vi "BRig_RT__Case_Exp__State_RewardPre__v11.vi"(0 "input_dataCurrent":u16[](array[numeric]), 7 "input_dataExp":u16[](array[numeric]), 9 "input_dataBlock":u16[][](array[numeric]), 11 "input_dataTrial":u16[][](array[numeric]), 12 "input_dataLC":u16[](array[numeric])) -> (1 "output_T_Reward":u16, 2 "output_c_nReward_total_R":u16, 3 "output_c_nReward_total_L":u16, 4 "output_dataCurrent":u16[](array[numeric]), 6 "output_DAB_L=L":bool, 8 "output_DAB_R=HighPorb":bool, 10 "output_dataBlock":u16[][](array[numeric]), 13 "output_c_nReward_total":u16, 14 "output_nReward":u16, 15 "output_dataTrial":u16[][](array[numeric]))   [LabVIEW 2014]
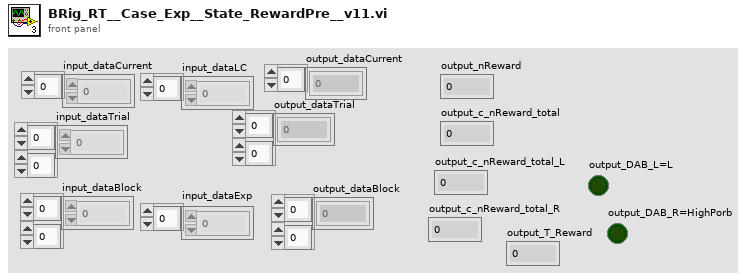
[diagram p1: front panel]
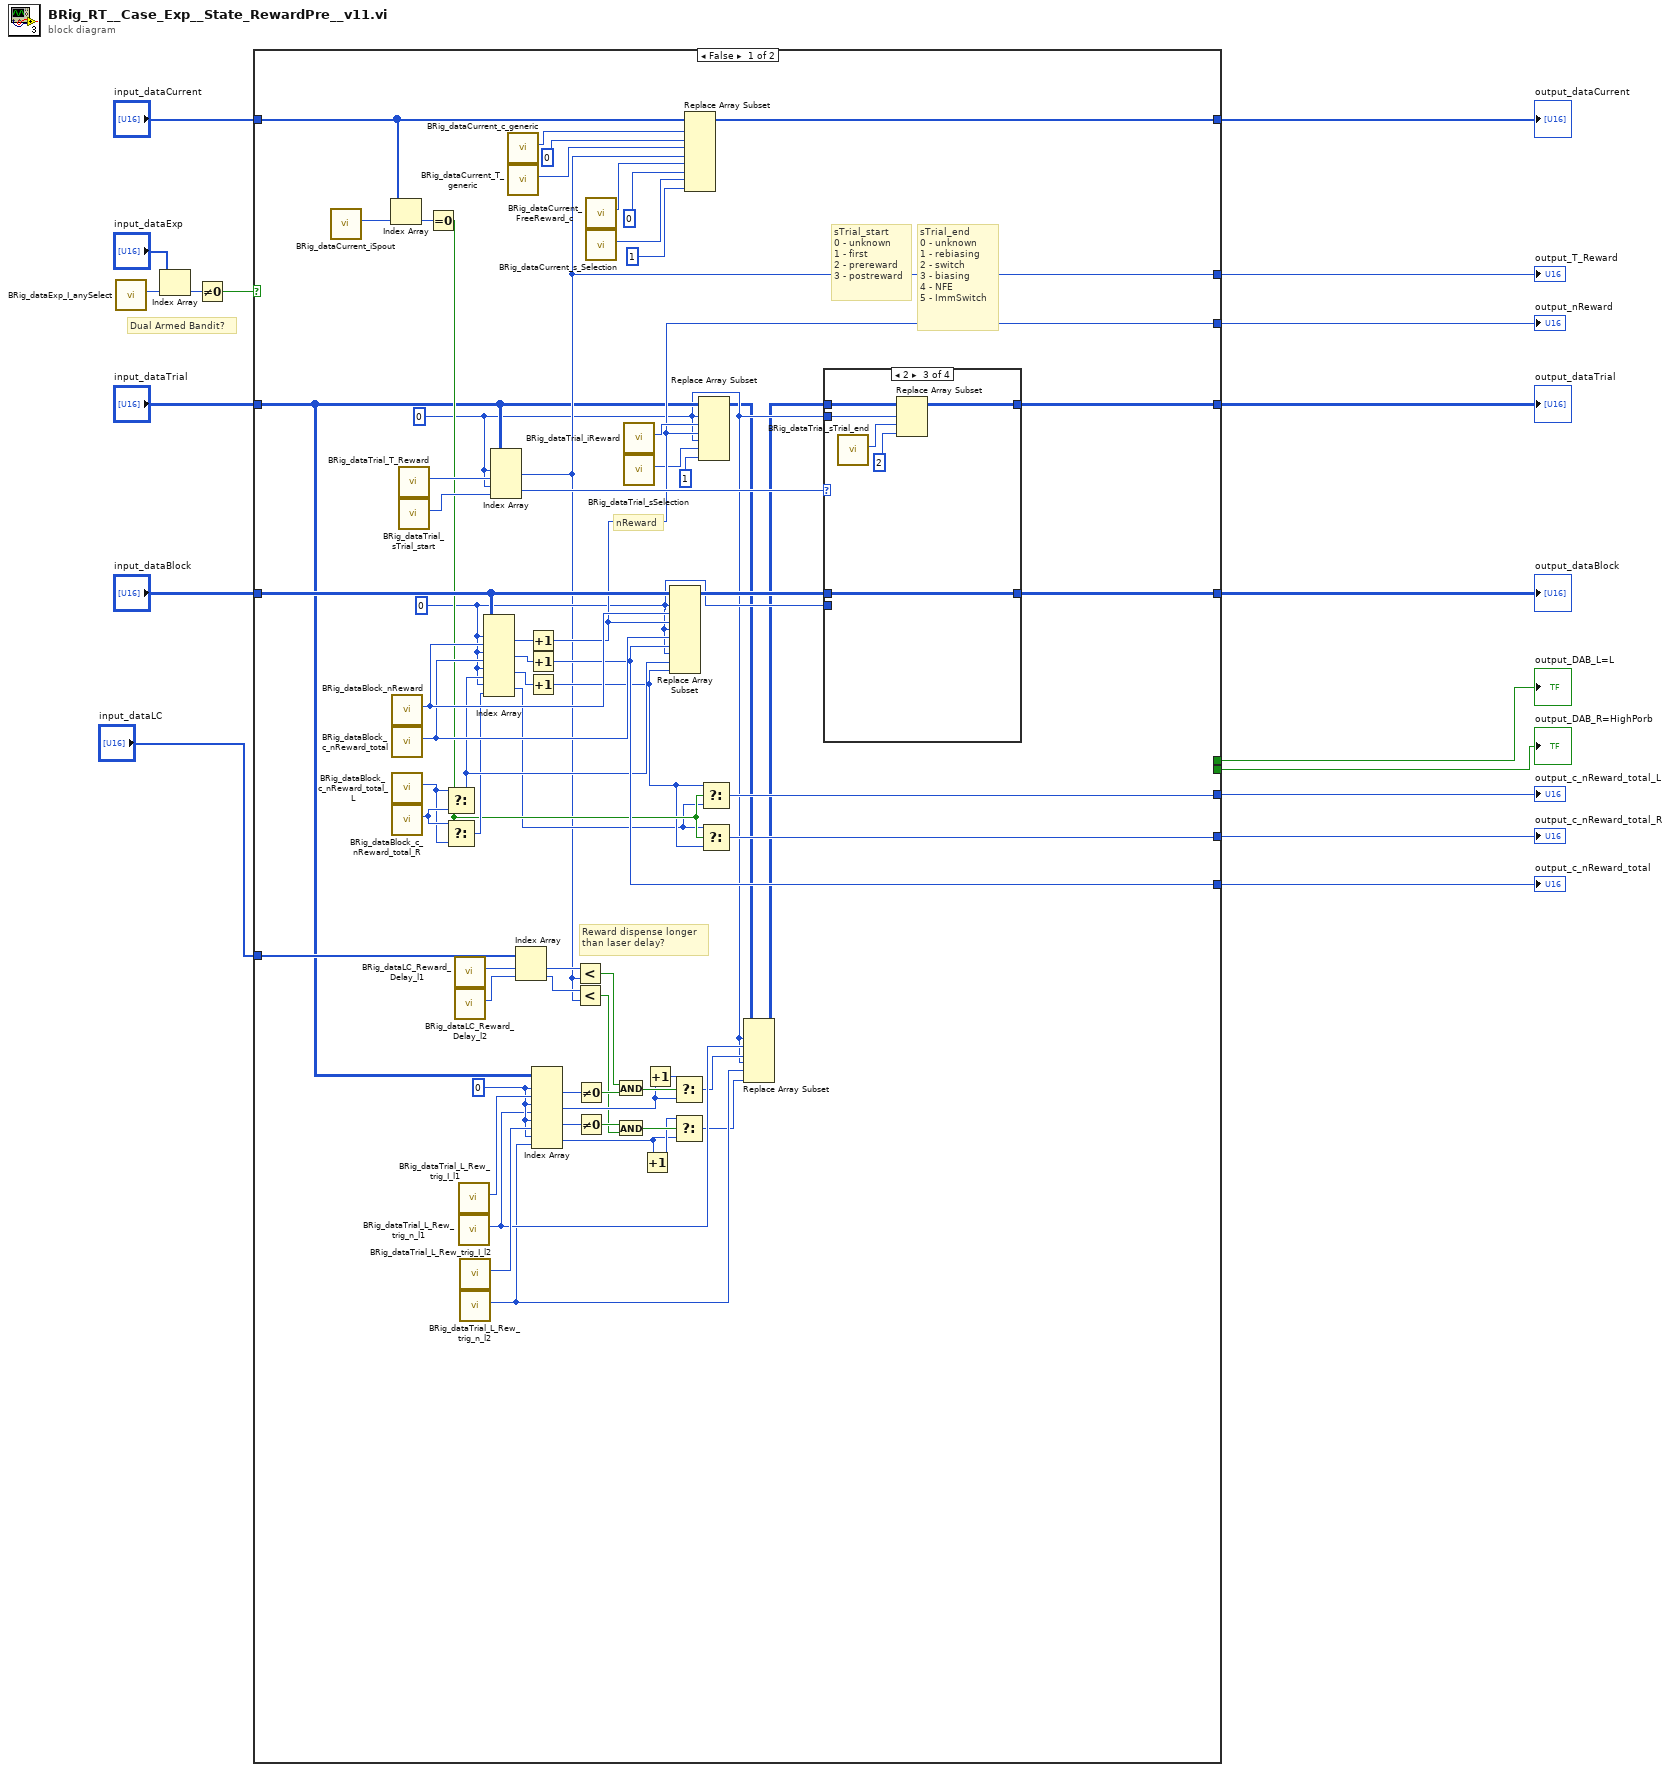
[diagram p0: block diagram]
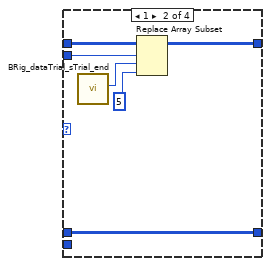
[diagram p3: hidden frame]
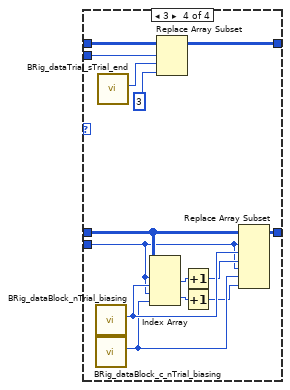
[diagram p4: hidden frame]
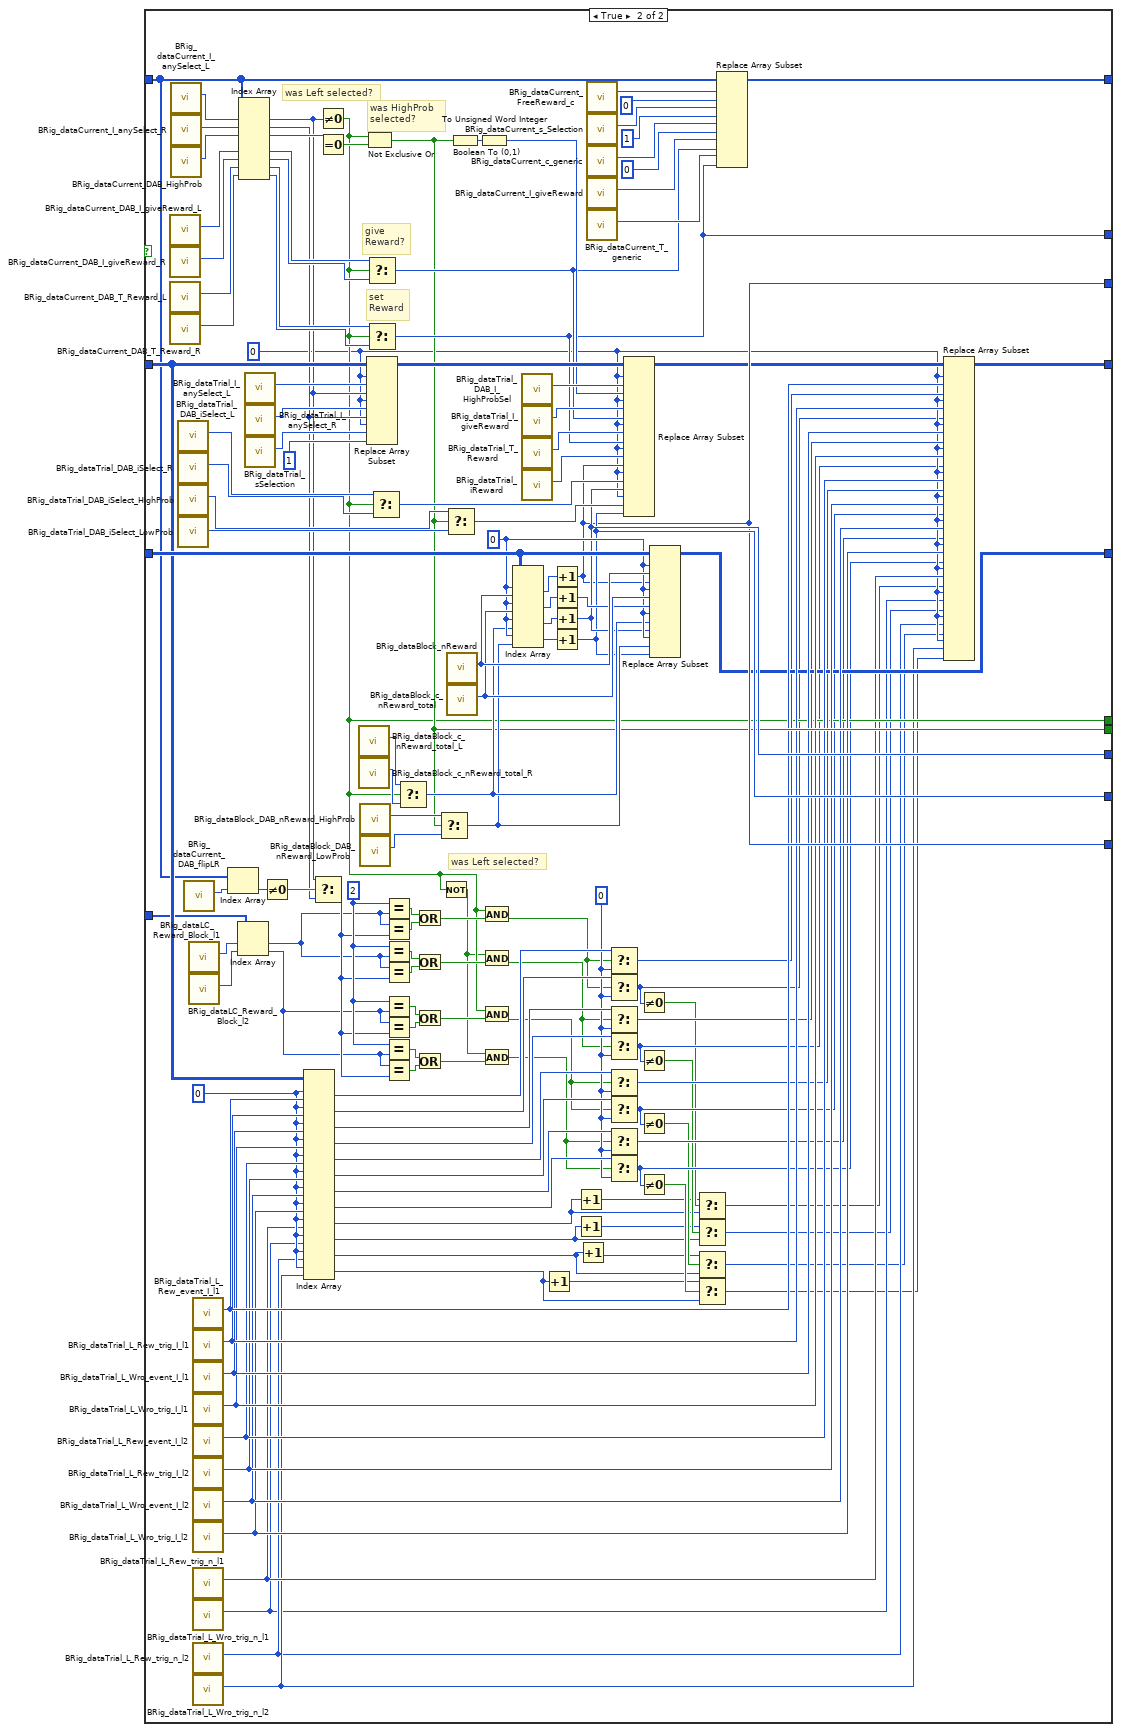
[diagram p5: hidden frame]
diagram:
  # "Dual Armed Bandit?"
  n1 = call "BRig_dataExp_I_anySelect.vi"() -> ("output_I_anySelect"=w13:i32)  [unwired: 11 in]
  n2 = Index Array(array="input_dataExp", index=w13) -> (element=w12:u16)
  n3 = Not Equal To 0?(x=w12) -> (x != 0?=w10:bool)
  n4 = case shown="False" w10 {
    tunnel: [w85 w255] -> w18
    tunnel: "input_dataCurrent" -> [w81 w192]
    tunnel: [w42 w200] -> w3
    tunnel: "input_dataBlock" -> [w79 w223]
    tunnel: [w74 w197] -> w17
    tunnel: "input_dataTrial" -> [w25 w195]
    tunnel: [w66 w197] -> w16
    tunnel: [w64 w167] -> w15
    tunnel: [w63 w175] -> w1
    tunnel: [w54 w199] -> w14
    tunnel: [w48 w198] -> w9
    tunnel: [_ w145] -> w5
    tunnel: [_ w196] -> w4
    tunnel: "input_dataLC" -> [w45 w194]
    frame False {
      w38 = 0 ("disabled index (row)")
      w24 = 0
      w49 = 0
      # "Reward dispense longer\nthan laser delay?"
      # "nReward"
      # "sTrial_end\n0 - unknown\n1 - rebiasing\n2 - switch\n3 - biasing\n4 - NFE\n5 - ImmSwitch"
      # "sTrial_start\n0 - unknown\n1 - first\n2 - prereward\n3 - postreward"
      n5 = call "BRig_dataCurrent_iSpout.vi"() -> ("output_iSpout"=w73:i32)  [unwired: 11 in]
      n6 = Index Array(array=w81, index=w73) -> (element=w72:u16)
      n7 = call "BRig_dataBlock_nReward.vi"() -> ("output_nReward"=w78:i32)  [unwired: 11 in]
      n8 = call "BRig_dataBlock_c_nReward_total.vi"() -> ("output_nReward_total"=w75:i32)  [unwired: 11 in]
      n9 = call "BRig_dataBlock_c_nReward_total_L.vi"() -> ("output_nReward_total_L"=w59:i32)  [unwired: 11 in]
      n10 = call "BRig_dataBlock_c_nReward_total_R.vi"() -> ("output_nReward_total_R"=w60:i32)  [unwired: 11 in]
      n11 = call "BRig_dataTrial_T_Reward.vi"() -> ("output_T_Reward"=w80:i32)  [unwired: 11 in]
      n12 = call "BRig_dataTrial_sTrial_start.vi"() -> ("output_sTrial_start"=w69:i32)  [unwired: 11 in]
      n13 = Equal To 0?(x=w72) -> (x = 0?=w57:bool)
      n14 = Select(t=w59, s=w57, f=w60) -> (s? t:f=w70:i32)
      n15 = Select(t=w60, s=w57, f=w59) -> (s? t:f=w58:i32)
      n16 = call "BRig_dataLC_Reward_Delay_l1.vi"() -> ("output_Reward_Delay"=w47:i32)  [unwired: 11 in]
      n17 = call "BRig_dataLC_Reward_Delay_l2.vi"() -> ("output_Reward_Delay_l2"=w46:i32)  [unwired: 11 in]
      n18 = call "BRig_dataTrial_L_Rew_trig_I_l1.vi"() -> ("output_L_Rew_trig_I_l1"=w41:i32)  [unwired: 11 in]
      n19 = call "BRig_dataTrial_L_Rew_trig_n_l1.vi"() -> ("output_L_Reward_trig_n_l1"=w32:i32)  [unwired: 11 in]
      n20 = call "BRig_dataTrial_L_Rew_trig_I_l2.vi"() -> ("output_L_Rew_trig_I_l2"=w39:i32)  [unwired: 11 in]
      n21 = call "BRig_dataTrial_L_Rew_trig_n_l2.vi"() -> ("output_L_Reward_trig_n_l2"=w27:i32)  [unwired: 11 in]
      n22 = Index Array(array=w79, index (row) #1=w49, index (col) #1=w78, index (row) #2=w49, index (col) #2=w75, index (row) #3=w49, index (col) #3=w70, index (row) #4=w49, index (col) #4=w58) -> (element #1=w77:u16, element #2=w76:u16, element #3=w71:u16, element #4=w55:u16)
      n23 = Index Array(array=w25, index (row) #1=w24, index (col) #1=w80, index (row) #2=w24, index (col) #2=w69) -> (element #1=w42:u16, element #2=w68:u16)
      n24 = call "BRig_dataCurrent_c_generic.vi"() -> ("output_count_generic"=w84:i32)  [unwired: 11 in]
      n25 = call "BRig_dataCurrent_T_generic.vi"() -> ("output_T_generic"=w83:i32)  [unwired: 11 in]
      n26 = Index Array(array=w45, index #1=w47, index #2=w46) -> (element #1=w44:u16, element #2=w43:u16)
      n27 = Increment(x=w77) -> (x+1=w66:u16)
      n28 = Increment(x=w76) -> (x+1=w74:u16)
      n29 = Increment(x=w71) -> (x+1=w56:u16)
      n30 = Index Array(array=w25, index (row) #1=w38, index (col) #1=w41, index (row) #2=w38, index (col) #2=w32, index (row) #3=w38, index (col) #3=w39, index (row) #4=w38, index (col) #4=w27) -> (element #1=w40:u16, element #2=w33:u16, element #3=w37:u16, element #4=w28:u16)
      n31 = Less?(x=w44, y=w42) -> (x < y?=w22:bool)
      n32 = Less?(x=w43, y=w42) -> (x < y?=w23:bool)
      n33 = Not Equal To 0?(x=w40) -> (x != 0?=w36:bool)
      n34 = Not Equal To 0?(x=w37) -> (x != 0?=w35:bool)
      n35 = call "BRig_dataCurrent_FreeReward_c.vi"() -> ("output_FreeReward_c"=w53:i32)  [unwired: 11 in]
      n36 = call "BRig_dataCurrent_s_Selection.vi"() -> ("output_s_Selection"=w51:i32)  [unwired: 11 in]
      n37 = And(x=w22, y=w36) -> (x .and. y?=w34:bool)
      n38 = And(x=w35, y=w23) -> (x .and. y?=w30:bool)
      n39 = call "BRig_dataTrial_iReward.vi"() -> ("output_iReward"=w67:i32)  [unwired: 11 in]
      n40 = call "BRig_dataTrial_sSelection.vi"() -> ("output_sSelection"=w62:i32)  [unwired: 11 in]
      n41 = Increment(x=w28) -> (x+1=w29:u16)
      n42 = Increment(x=w33) -> (x+1=w19:u16)
      n43 = Replace Array Subset(array=w79, new element #1=w66, index (row) #1=w49, index (col) #1=w78, new element #2=w74, index (row) #2=w49, index (col) #2=w75, new element #3=w56, index (row) #3=w49, index (col) #3=w70) -> (w65:u16[][])
      n44 = Select(t=w19, s=w34, f=w33) -> (s? t:f=w31:u16)
      n45 = Select(t=w29, s=w30, f=w28) -> (s? t:f=w26:u16)
      n46 = Replace Array Subset(array=w81, new element #1=u16 0 ("new element/subarray"), index #1=w84, new element #2=w42, index #2=w83, new element #3=u16 0 ("new element/subarray"), index #3=w53, new element #4=u16 1 ("new element/subarray"), index #4=w51) -> (w85:u16[])
      n47 = Replace Array Subset(array=w25, new element #1=w66, index (row) #1=w24, index (col) #1=w67, new element #2=u16 1 ("new element/subarray"), index (row) #2=w24, index (col) #2=w62) -> (w21:u16[][])
      n48 = Select(t=w56, s=w57, f=w55) -> (s? t:f=w54:u16)
      n49 = Select(t=w55, s=w57, f=w56) -> (s? t:f=w48:u16)
      n50 = Replace Array Subset(array=w21, new element #1=w31, index (row) #1=w24, index (col) #1=w32, new element #2=w26, index (row) #2=w24, index (col) #2=w27) -> (w20:u16[][])
      n51 = case shown="2" w68 {
        tunnel: w20 -> [w87 w93 w99 w113]
        tunnel: w24 -> [_ w91 w97 w111]
        tunnel: [w87 w92 w98 w112] -> w63
        tunnel: w65 -> [w86 w88 w94 w107]
        tunnel: [w86 w88 w94 w108] -> w64
        tunnel: w49 -> [_ _ _ w103]
        frame 0, Default {
        }
        frame 1 {
          n52 = call "BRig_dataTrial_sTrial_end.vi"() -> ("output_sTrial_end"=w90:i32)  [unwired: 11 in]
          n53 = Replace Array Subset(array=w93, new element=u16 5 ("new element/subarray"), index (row)=w91, index (col)=w90) -> (w92:u16[][])
        }
        frame 2 {
          n54 = call "BRig_dataTrial_sTrial_end.vi"() -> ("output_sTrial_end"=w96:i32)  [unwired: 11 in]
          n55 = Replace Array Subset(array=w99, new element=u16 2 ("new element/subarray"), index (row)=w97, index (col)=w96) -> (w98:u16[][])
        }
        frame 3 {
          n56 = call "BRig_dataBlock_nTrial_biasing.vi"() -> ("output_nTrial_biasing"=w106:i32)  [unwired: 11 in]
          n57 = call "BRig_dataBlock_c_nTrial_biasing.vi"() -> ("output_c_nTrial_biasing"=w101:i32)  [unwired: 11 in]
          n58 = call "BRig_dataTrial_sTrial_end.vi"() -> ("output_sTrial_end"=w110:i32)  [unwired: 11 in]
          n59 = Index Array(array=w107, index (row) #1=w103, index (col) #1=w106, index (row) #2=w103, index (col) #2=w101) -> (element #1=w105:u16, element #2=w102:u16)
          n60 = Replace Array Subset(array=w113, new element=u16 3 ("new element/subarray"), index (row)=w111, index (col)=w110) -> (w112:u16[][])
          n61 = Increment(x=w105) -> (x+1=w104:u16)
          n62 = Increment(x=w102) -> (x+1=w100:u16)
          n63 = Replace Array Subset(array=w107, new element #1=w104, index (row) #1=w103, index (col) #1=w106, new element #2=w100, index (row) #2=w103, index (col) #2=w101) -> (w108:u16[][])
        }
      }
    }
    frame True {
      w157 = u16 0 ("f")
      w178 = u16 2 ("y")
      w140 = 0 ("index (row)")
      w221 = 0
      w138 = 0
      # "was Left selected?"
      # "set\nReward"
      # "give\nReward?"
      # "was HighProb\nselected?"
      # "was Left selected?"
      n64 = call "BRig_dataCurrent_DAB_I_giveReward_L.vi"() -> ("output_DAB_I_giveReward_L"=w241:i32)  [unwired: 11 in]
      n65 = call "BRig_dataCurrent_DAB_I_giveReward_R.vi"() -> ("output_DAB_I_giveReward_R"=w240:i32)  [unwired: 11 in]
      n66 = call "BRig_dataCurrent_DAB_T_Reward_L.vi"() -> ("output_DAB_T_Reward_L"=w235:i32)  [unwired: 11 in]
      n67 = call "BRig_dataCurrent_DAB_T_Reward_R.vi"() -> ("output_DAB_T_Reward_R"=w234:i32)  [unwired: 11 in]
      n68 = call "BRig_dataCurrent_I_anySelect_L.vi"() -> ("output_IanySelect_L"=w246:i32)  [unwired: 11 in]
      n69 = call "BRig_dataCurrent_I_anySelect_R.vi"() -> ("output_IanySelect_R"=w245:i32)  [unwired: 11 in]
      n70 = call "BRig_dataCurrent_DAB_HighProb.vi"() -> ("output_DAB_HighProb"=w244:i32)  [unwired: 11 in]
      n71 = call "BRig_dataTrial_DAB_iSelect_L.vi"() -> ("output_DAB_iSelect_L"=w212:i32)  [unwired: 11 in]
      n72 = call "BRig_dataTrial_DAB_iSelect_R.vi"() -> ("output_DAB_iSelect_R"=w211:i32)  [unwired: 11 in]
      n73 = call "BRig_dataTrial_DAB_iSelect_HighProb.vi"() -> ("output_DAB_iSelect_HighProb"=w209:i32)  [unwired: 11 in]
      n74 = call "BRig_dataTrial_DAB_iSelect_LowProb.vi"() -> ("output_DAB_iSelect_LowProb"=w210:i32)  [unwired: 11 in]
      n75 = call "BRig_dataCurrent_DAB_flipLR.vi"() -> ("output_DAB_flipLR"=w191:i32)  [unwired: 11 in]
      n76 = call "BRig_dataLC_Reward_Block_l1.vi"() -> ("output_Reward_Block"=w193:i32)  [unwired: 11 in]
      n77 = call "BRig_dataLC_Reward_Block_l2.vi"() -> ("output_Reward_Block_l2"=w153:i32)  [unwired: 11 in]
      n78 = call "BRig_dataTrial_L_Rew_event_I_l1.vi"() -> ("output_L_Rew_event_I_l1"=w174:i32)  [unwired: 11 in]
      n79 = call "BRig_dataTrial_L_Rew_trig_I_l1.vi"() -> ("output_L_Rew_trig_I_l1"=w173:i32)  [unwired: 11 in]
      n80 = call "BRig_dataTrial_L_Wro_event_I_l1.vi"() -> ("output_L_Wro_event_I_l1"=w172:i32)  [unwired: 11 in]
      n81 = call "BRig_dataTrial_L_Wro_trig_I_l1.vi"() -> ("output_L_Wro_trig_I_l1"=w171:i32)  [unwired: 11 in]
      n82 = call "BRig_dataTrial_L_Rew_event_I_l2.vi"() -> ("output_L_Rew_event_I_l2"=w170:i32)  [unwired: 11 in]
      n83 = call "BRig_dataTrial_L_Rew_trig_I_l2.vi"() -> ("output_L_Rew_trig_I_l2"=w169:i32)  [unwired: 11 in]
      n84 = call "BRig_dataTrial_L_Wro_event_I_l2.vi"() -> ("output_L_Wro_event_I_l2"=w168:i32)  [unwired: 11 in]
      n85 = call "BRig_dataTrial_L_Wro_trig_I_l2.vi"() -> ("output_L_Wro_trig_I_l2"=w166:i32)  [unwired: 11 in]
      n86 = call "BRig_dataTrial_L_Rew_trig_n_l1.vi"() -> ("output_L_Reward_trig_n_l1"=w139:i32)  [unwired: 11 in]
      n87 = call "BRig_dataTrial_L_Wro_trig_n_l1.vi"() -> ("output_L_Wrong_trig_n_l1"=w127:i32)  [unwired: 11 in]
      n88 = call "BRig_dataTrial_L_Rew_trig_n_l2.vi"() -> ("output_L_Reward_trig_n_l2"=w128:i32)  [unwired: 11 in]
      n89 = call "BRig_dataTrial_L_Wro_trig_n_l2.vi"() -> ("output_L_Wrong_trig_n_l2"=w137:i32)  [unwired: 11 in]
      n90 = Index Array(array=w192, index=w191) -> (element=w190:u16)
      n91 = Index Array(array=w194, index #1=w193, index #2=w153) -> (element #1=w151:u16, element #2=w152:u16)
      n92 = Index Array(array=w192, index #1=w246, index #2=w245, index #3=w244, index #5=w241, index #6=w240, index #7=w235, index #8=w234) -> (element #1=w188:u16, element #2=w187:u16, element #3=w243:u16, element #5=w239:u16, element #6=w238:u16, element #7=w237:u16, element #8=w236:u16)  [unwired: 1 in, 1 out]
      n93 = call "BRig_dataTrial_I_anySelect_L.vi"() -> ("output_I_allReward_L"=w233:i32)  [unwired: 11 in]
      n94 = call "BRig_dataTrial_I_anySelect_R.vi"() -> ("output_I_anySelect_R"=w232:i32)  [unwired: 11 in]
      n95 = call "BRig_dataTrial_sSelection.vi"() -> ("output_sSelection"=w231:i32)  [unwired: 11 in]
      n96 = Not Equal To 0?(x=w190) -> (x != 0?=w189:bool)
      n97 = Index Array(array=w195, index (row) #1=w140, index (col) #1=w174, index (row) #2=w140, index (col) #2=w173, index (row) #3=w140, index (col) #3=w172, index (row) #4=w140, index (col) #4=w171, index (row) #5=w140, index (col) #5=w170, index (row) #6=w140, index (col) #6=w169, index (row) #7=w140, index (col) #7=w168, index (row) #8=w140, index (col) #8=w166, index (row) #9=w140, index (col) #9=w139, index (row) #10=w140, index (col) #10=w127, index (row) #11=w140, index (col) #11=w128, index (row) #12=w140, index (col) #12=w137) -> (element #1=w165:u16, element #2=w164:u16, element #3=w163:u16, element #4=w162:u16, element #5=w161:u16, element #6=w160:u16, element #7=w159:u16, element #8=w158:u16, element #9=w124:u16, element #10=w122:u16, element #11=w120:u16, element #12=w118:u16)
      n98 = Select(t=w188, s=w189, f=w187) -> (s? t:f=w177:u16)
      n99 = Not Equal To 0?(x=w188) -> (x != 0?=w145:bool)
      n100 = Equal To 0?(x=w243) -> (x = 0?=w242:bool)
      n101 = call "BRig_dataBlock_c_nReward_total_L.vi"() -> ("output_nReward_total_L"=w220:i32)  [unwired: 11 in]
      n102 = call "BRig_dataBlock_c_nReward_total_R.vi"() -> ("output_nReward_total_R"=w219:i32)  [unwired: 11 in]
      n103 = call "BRig_dataBlock_DAB_nReward_HighProb.vi"() -> ("output_DAB_nReward_HighProb"=w218:i32)  [unwired: 11 in]
      n104 = call "BRig_dataBlock_DAB_nReward_LowProb.vi"() -> ("output_DAB_nReward_LowProb"=w217:i32)  [unwired: 11 in]
      n105 = Not Exclusive Or(1:w242, 2:w145) -> (0:w196:bool)
      n106 = Select(t=w239, s=w145, f=w238) -> (s? t:f=w201:u16)
      n107 = Select(t=w237, s=w145, f=w236) -> (s? t:f=w200:u16)
      n108 = Replace Array Subset(array=w195, new element #1=w188, index (row) #1=w138, index (col) #1=w233, new element #2=w187, index (row) #2=w138, index (col) #2=w232, new element #3=u16 1 ("new element/subarray"), index (row) #3=w138, index (col) #3=w231) -> (w229:u16[][])
      n109 = Select(t=w212, s=w145, f=w211) -> (s? t:f=w207:i32)
      n110 = Equal?(x=w178, y=w151) -> (x = y?=w186:bool)
      n111 = Equal?(x=w151, y=w177) -> (x = y?=w185:bool)
      n112 = Equal?(x=w178, y=w151) -> (x = y?=w184:bool)
      n113 = Equal?(x=w151, y=w177) -> (x = y?=w183:bool)
      n114 = Equal?(x=w178, y=w152) -> (x = y?=w182:bool)
      n115 = Equal?(x=w152, y=w177) -> (x = y?=w181:bool)
      n116 = Equal?(x=w178, y=w152) -> (x = y?=w179:bool)
      n117 = Equal?(x=w152, y=w177) -> (x = y?=w180:bool)
      n118 = Select(t=w220, s=w145, f=w219) -> (s? t:f=w214:i32)
      n119 = Or(x=w186, y=w185) -> (x .or. y?=w150:bool)
      n120 = Or(x=w184, y=w183) -> (x .or. y?=w148:bool)
      n121 = Or(x=w182, y=w181) -> (x .or. y?=w146:bool)
      n122 = Or(x=w179, y=w180) -> (x .or. y?=w142:bool)
      n123 = Select(t=w218, s=w196, f=w217) -> (s? t:f=w213:i32)
      n124 = Not(x=w145) -> (.not. x?=w143:bool)
      n125 = Select(t=w209, s=w196, f=w210) -> (s? t:f=w208:i32)
      n126 = call "BRig_dataBlock_nReward.vi"() -> ("output_nReward"=w228:i32)  [unwired: 11 in]
      n127 = call "BRig_dataBlock_c_nReward_total.vi"() -> ("output_nReward_total"=w225:i32)  [unwired: 11 in]
      n128 = Boolean To (0,1)(Boolean=w196) -> (0, 1=w222:i16)
      n129 = To Unsigned Word Integer(number=w222) -> (unsigned 16bit integer=w202:u16)
      n130 = And(x=w145, y=w150) -> (x .and. y?=w149:bool)
      n131 = And(x=w143, y=w148) -> (x .and. y?=w147:bool)
      n132 = And(x=w145, y=w146) -> (x .and. y?=w144:bool)
      n133 = And(x=w143, y=w142) -> (x .and. y?=w141:bool)
      n134 = Index Array(array=w223, index (row) #1=w221, index (col) #1=w228, index (row) #2=w221, index (col) #2=w225, index (row) #3=w221, index (col) #3=w214, index (row) #4=w221, index (col) #4=w213) -> (element #1=w227:u16, element #2=w226:u16, element #3=w216:u16, element #4=w215:u16)
      n135 = call "BRig_dataTrial_DAB_I_HighProbSel.vi"() -> ("output_DAB_I_HighProbSel"=w203:i32)  [unwired: 11 in]
      n136 = call "BRig_dataTrial_I_giveReward.vi"() -> ("output_I_giveReward"=w204:i32)  [unwired: 11 in]
      n137 = call "BRig_dataTrial_T_Reward.vi"() -> ("output_T_Reward"=w205:i32)  [unwired: 11 in]
      n138 = call "BRig_dataTrial_iReward.vi"() -> ("output_iReward"=w206:i32)  [unwired: 11 in]
      n139 = Increment(x=w118) -> (x+1=w119:u16)
      n140 = Increment(x=w227) -> (x+1=w197:u16)
      n141 = Increment(x=w226) -> (x+1=w224:u16)
      n142 = Increment(x=w216) -> (x+1=w199:u16)
      n143 = Increment(x=w215) -> (x+1=w198:u16)
      n144 = Increment(x=w124) -> (x+1=w125:u16)
      n145 = Increment(x=w122) -> (x+1=w123:u16)
      n146 = Increment(x=w120) -> (x+1=w121:u16)
      n147 = call "BRig_dataCurrent_FreeReward_c.vi"() -> ("output_FreeReward_c"=w254:i32)  [unwired: 11 in]
      n148 = call "BRig_dataCurrent_s_Selection.vi"() -> ("output_s_Selection"=w252:i32)  [unwired: 11 in]
      n149 = call "BRig_dataCurrent_c_generic.vi"() -> ("output_count_generic"=w250:i32)  [unwired: 11 in]
      n150 = call "BRig_dataCurrent_I_giveReward.vi"() -> ("output_I_giveReward"=w248:i32)  [unwired: 11 in]
      n151 = call "BRig_dataCurrent_T_generic.vi"() -> ("output_T_generic"=w247:i32)  [unwired: 11 in]
      n152 = Select(t=w165, s=w149, f=w157) -> (s? t:f=w154:u16)
      n153 = Select(t=w164, s=w149, f=w157) -> (s? t:f=w136:u16)
      n154 = Select(t=w163, s=w147, f=w157) -> (s? t:f=w155:u16)
      n155 = Select(t=w162, s=w147, f=w157) -> (s? t:f=w135:u16)
      n156 = Select(t=w161, s=w144, f=w157) -> (s? t:f=w156:u16)
      n157 = Select(t=w160, s=w144, f=w157) -> (s? t:f=w133:u16)
      n158 = Select(t=w159, s=w141, f=w157) -> (s? t:f=w134:u16)
      n159 = Select(t=w158, s=w141, f=w157) -> (s? t:f=w132:u16)
      n160 = Replace Array Subset(array=w229, new element #1=w202, index (row) #1=w138, index (col) #1=w203, new element #2=w201, index (row) #2=w138, index (col) #2=w204, new element #3=w200, index (row) #3=w138, index (col) #3=w205, new element #4=w197, index (row) #4=w138, index (col) #4=w206, new element #5=w199, index (row) #5=w138, index (col) #5=w207, new element #6=w198, index (row) #6=w138, index (col) #6=w208) -> (w176:u16[][])
      n161 = Not Equal To 0?(x=w136) -> (x != 0?=w131:bool)
      n162 = Not Equal To 0?(x=w135) -> (x != 0?=w130:bool)
      n163 = Not Equal To 0?(x=w133) -> (x != 0?=w129:bool)
      n164 = Not Equal To 0?(x=w132) -> (x != 0?=w126:bool)
      n165 = Replace Array Subset(array=w223, new element #1=w197, index (row) #1=w221, index (col) #1=w228, new element #2=w224, index (row) #2=w221, index (col) #2=w225, new element #3=w199, index (row) #3=w221, index (col) #3=w214, new element #4=w198, index (row) #4=w221, index (col) #4=w213) -> (w167:u16[][])
      n166 = Select(t=w125, s=w131, f=w124) -> (s? t:f=w117:u16)
      n167 = Select(t=w123, s=w130, f=w122) -> (s? t:f=w116:u16)
      n168 = Select(t=w121, s=w129, f=w120) -> (s? t:f=w115:u16)
      n169 = Select(t=w119, s=w126, f=w118) -> (s? t:f=w114:u16)
      n170 = Replace Array Subset(array=w192, new element #1=u16 0 ("new element/subarray"), index #1=w254, new element #2=u16 1 ("new element/subarray"), index #2=w252, new element #3=u16 0 ("new element/subarray"), index #3=w250, new element #4=w201, index #4=w248, new element #5=w200, index #5=w247) -> (w255:u16[])
      n171 = Replace Array Subset(array=w176, new element #1=w154, index (row) #1=w138, index (col) #1=w174, new element #2=w136, index (row) #2=w138, index (col) #2=w173, new element #3=w155, index (row) #3=w138, index (col) #3=w172, new element #4=w135, index (row) #4=w138, index (col) #4=w171, new element #5=w156, index (row) #5=w138, index (col) #5=w170, new element #6=w133, index (row) #6=w138, index (col) #6=w169, new element #7=w134, index (row) #7=w138, index (col) #7=w168, new element #8=w132, index (row) #8=w138, index (col) #8=w166, new element #9=w117, index (row) #9=w138, index (col) #9=w139, new element #10=w116, index (row) #10=w138, index (col) #10=w127, new element #11=w115, index (row) #11=w138, index (col) #11=w128, new element #12=w114, index (row) #12=w138, index (col) #12=w137) -> (w175:u16[][])
    }
  }
  "output_dataCurrent" <- w18
  "output_dataBlock" <- w15
  "output_dataTrial" <- w1
  "output_nReward" <- w16
  "output_c_nReward_total" <- w17
  "output_c_nReward_total_L" <- w14
  "output_c_nReward_total_R" <- w9
  "output_T_Reward" <- w3
  "output_DAB_L=L" <- w5
  "output_DAB_R=HighPorb" <- w4
